vi "Timer_Logger.vi"(0 "Wait_Time":u32=10, 11 "Error_In":errorcluster, 13 "Timer_Select":T1=enum."Time_Out?") -> (4 "Time_Out?":bool, 15 "Error_Out":errorcluster)   [LabVIEW 2021]
doc: "Used for time out opertion of logger."
uses:
  Controls/Timer_Data.ctl
  Controls/Timer_Select.ctl
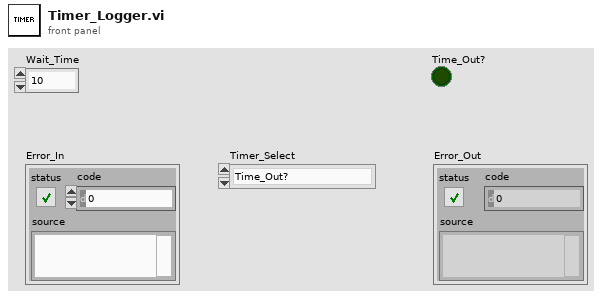
[diagram p1: front panel]
types:
  T1 = typedef "Timer_Select.ctl" = enum16{"Start_Timer", "Time_Out?", "Stop_Timer"}
  T2 = typedef "Timer_Data.ctl" = cluster{"Start_Time":dbl, "Start?":bool, "Wait_Time":dbl}
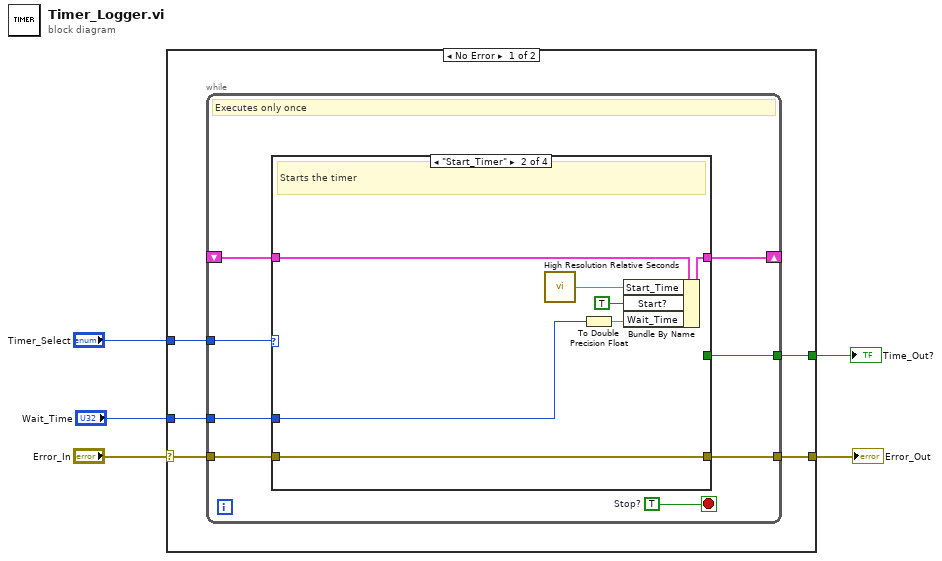
[diagram p0: block diagram]
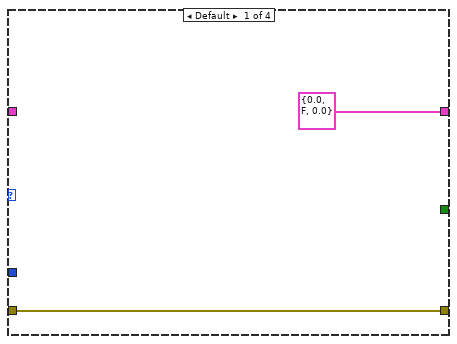
[diagram p2: hidden frame]
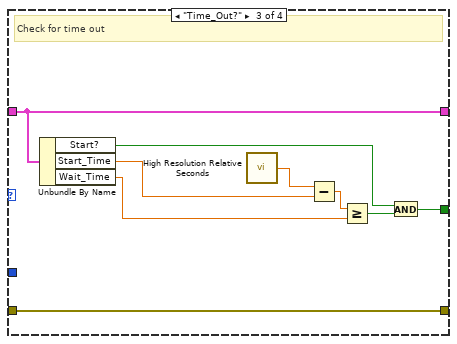
[diagram p3: hidden frame]
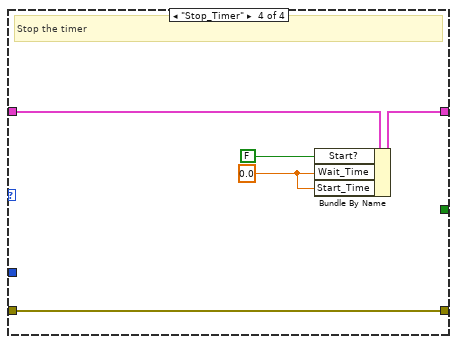
[diagram p4: hidden frame]
diagram:
  n1 = case shown="No Error" "Error_In" {
    selector: "Error_In" -> [w6 w42]
    tunnel: [w10 _] -> w5
    tunnel: [w9 w42] -> w4
    tunnel: "Wait_Time" -> [w8 _]
    tunnel: "Timer_Select" -> [w7 _]
    frame No Error {
      n2 = while {
        tunnel: w7 -> [w18]
        shift-right: [w17] -> _
        shift-left: _ -> [w16]
        tunnel: [w15] -> w10
        tunnel: w6 -> [w13]
        tunnel: [w12] -> w9
        tunnel: w8 -> [w11]
        stop <- w14 stop-if-true
        w14 = TRUE  # Stop?
        # "Executes only once"
        n3 = case shown="\"Start_Timer\"" w18 {
          tunnel: [T2 {"Start_Time"=0.0, "Start?"=FALSE, "Wait_Time"=0.0} ("Cluster") w25 w31 w39] -> w17
          tunnel: w16 -> [_ w26 w31 w40]
          tunnel: [_ _ w32 _] -> w15
          tunnel: w13 -> [w20 w27 w34 w41]
          tunnel: [w20 w27 w34 w41] -> w12
          tunnel: w11 -> [_ w22 _ _]
          frame Default {
          }
          frame "Start_Timer" {
            # "Starts the timer"
            n4 = call <vilib>:"High Resolution Relative Seconds.vi"() -> ("relative seconds"=w24:dbl)
            n5 = To Double Precision Float(number=w22) -> (double precision float=w21:dbl)
            n6 = Bundle By Name(cluster=w26, "Start_Time"=w24, "Start?"=TRUE, "Wait_Time"=w21) -> (w25:T2)
          }
          frame "Time_Out?" {
            # "Check for time out"
            n7 = Unbundle By Name(w31) -> ("Start?"=w29:bool, "Start_Time"=w30:dbl, "Wait_Time"=w28:dbl)
            n8 = call <vilib>:"High Resolution Relative Seconds.vi"() -> ("relative seconds"=w33:dbl)
            n9 = Subtract(x=w33, y=w30) -> (x-y=w36:dbl)
            n10 = Greater Or Equal?(x=w36, y=w28) -> (x >= y?=w35:bool)
            n11 = And(x=w29, y=w35) -> (x .and. y?=w32:bool)
          }
          frame "Stop_Timer" {
            w37 = 0.0 ("Wait_Time")
            # "Stop the timer"
            n12 = Bundle By Name(cluster=w40, "Start?"=FALSE, "Wait_Time"=w37, "Start_Time"=w37) -> (w39:T2)
          }
        }
      }
    }
    frame Error {
    }
  }
  "Time_Out?" <- w5
  "Error_Out" <- w4
